vi "Initialize Sync Stuff.vi"(8 "error in (no error)":errorcluster, 11 "IP Connection in":refnum<class "IP Connection.lvclass">) -> (0 "error out":errorcluster, 3 "IP Connection out":refnum<class "IP Connection.lvclass">)   [LabVIEW 2011, in "Tinkerforge.lvlib" / "IP Connection.lvclass"]
doc: "This VI initializes the synchronization stuff."
uses:
  IP Connection.lvclass
  Device/Device.lvclass
  Type Definitions/Enumerate CB.ctl
  Type Definitions/Answer.ctl
  Type Definitions/Request Type.ctl
  Type Definitions/Request Identifier.ctl
  Type Definitions/Message.ctl
  IP Connection.lvclass/IP Connection.ctl
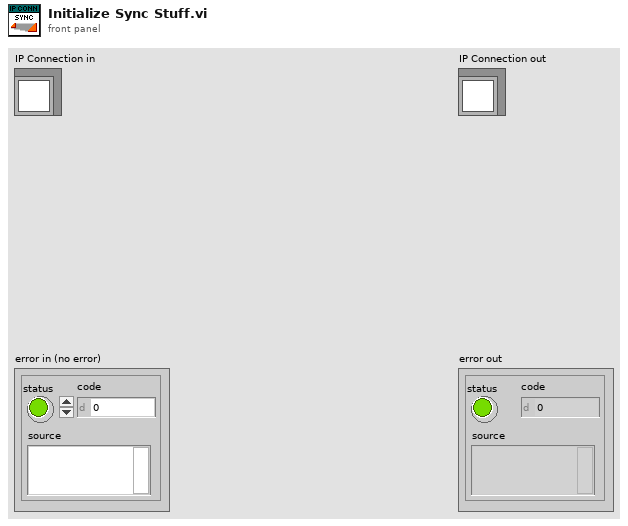
[diagram p1: front panel]
types:
  T1 = typedef "Tinkerforge.lvlib/IP Connection.lvclass/Enumerate CB.ctl" = cluster{"UID":string, "Name":string, "Stack ID":u8, "is new?":bool}
  T2 = typedef "Tinkerforge.lvlib/IP Connection.lvclass/Answer.ctl" = cluster{"Request GUID":string, "Request Type":T3, "Sucessful":bool, "Data":variant, "Error":errorcluster}
  T3 = typedef "Tinkerforge.lvlib/IP Connection.lvclass/Request Type.ctl" = enum8{"Invalid", "Write"}
  T4 = typedef "Tinkerforge.lvlib/IP Connection.lvclass/Message.ctl" = cluster{"Stack ID":u8, "Function ID":u8, "Data":string, "Request GUID":string, "Timeout":i32, "Response":bool}
  T5 = typedef "Tinkerforge.lvlib/IP Connection.lvclass/Request Identifier.ctl" = cluster{"Stack ID":u8, "Function ID":u8, "Request GUID":string, "Remaining Timeout":i32}
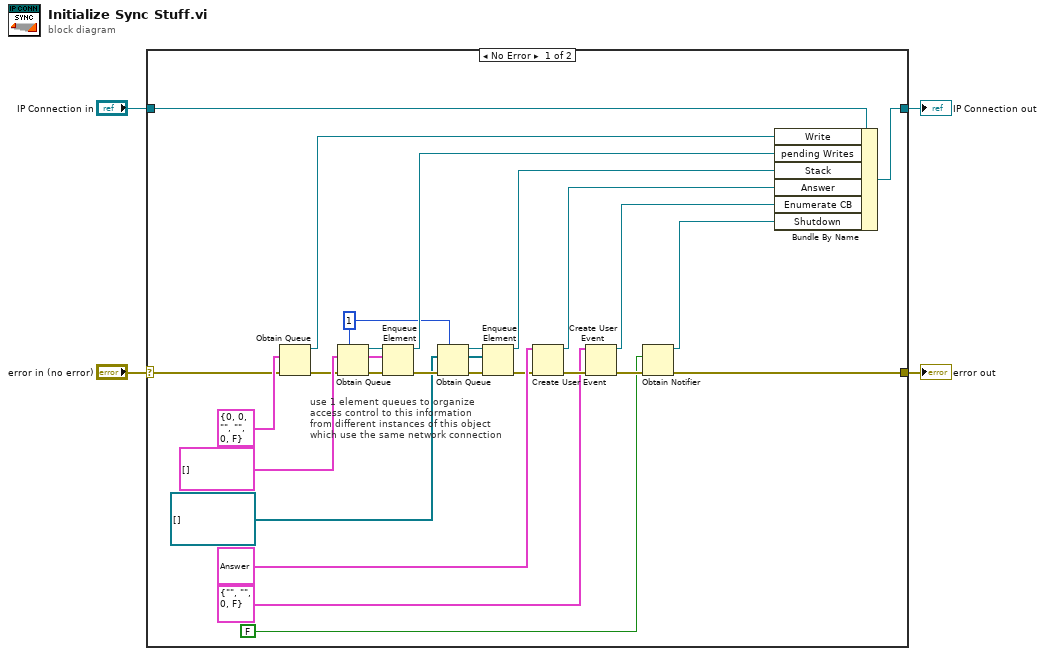
[diagram p0: block diagram]
diagram:
  n1 = case shown="No Error" "error in (no error)" {
    selector: "error in (no error)" -> [w9 w32]
    tunnel: [w7 w32] -> w3
    tunnel: [w28 w31] -> w1
    tunnel: "IP Connection in" -> [w29 w31]
    frame No Error {
      w12 = refnum<class "Device.lvclass">[] []
      w14 = 1 ("max queue size (-1, unlimited)")
      w24 = T5[] []
      # "use 1 element queues to organize\naccess control to this information\nfrom different instances of this object\nwhich use the same network connection"
      n2 = Obtain Queue(element data type=T4 {"Stack ID"=0, "Function ID"=0, "Data"="", "Request GUID"="", "Timeout"=0, "Response"=FALSE} ("Write Data"), error in (no error)=w9) -> (queue out=w27:refnum<queue>, error out=w20:errorcluster)  [unwired: 3 in, 1 out]
      n3 = Obtain Queue(max queue size (-1, unlimited)=w14, element data type=w24, error in (no error)=w20) -> (queue out=w25:refnum<queue>, error out=w26:errorcluster)  [unwired: 2 in, 1 out]
      n4 = Enqueue Element(queue=w25, element=w24, error in (no error)=w26) -> (queue out=w23:refnum<queue>, error out=w15:errorcluster)  [unwired: 1 in, 1 out]
      n5 = Obtain Queue(max queue size (-1, unlimited)=w14, element data type=w12, error in (no error)=w15) -> (queue out=w13:refnum<queue>, error out=w16:errorcluster)  [unwired: 2 in, 1 out]
      n6 = Enqueue Element(queue=w13, element=w12, error in (no error)=w16) -> (queue out=w10:refnum<queue>, error out=w11:errorcluster)  [unwired: 1 in, 1 out]
      n7 = Create User Event(user event datatype=T2 {"Request GUID"="", "Request Type"=enum."Invalid", "Sucessful"=FALSE, "Data"=variant, "Error"={"status"=FALSE, "code"=0, "source"=""}} ("Answer"), error in=w11) -> (user event=w21:refnum<user-event>, error out=w19:errorcluster)
      n8 = Create User Event(user event datatype=T1 {"UID"="", "Name"="", "Stack ID"=0, "is new?"=FALSE} ("Enumerate CB"), error in=w19) -> (user event=w17:refnum<user-event>, error out=w8:errorcluster)
      n9 = Obtain Notifier(notification data type=FALSE, error in (no error)=w8) -> (notifier out=w5:refnum<notifier>, error out=w7:errorcluster)  [unwired: 2 in, 1 out]
      n10 = Bundle By Name(cluster=w29, "Write"=w27, "pending Writes"=w23, "Stack"=w10, "Answer"=w21, "Enumerate CB"=w17, "Shutdown"=w5) -> (w28:refnum<class "IP Connection.lvclass">)
    }
    frame Error {
    }
  }
  "error out" <- w3
  "IP Connection out" <- w1
